vi "Image Transmission.vi"() -> ()   [LabVIEW 2013]
uses:
  <vilib>/picture/picture.llb/Draw True-Color Pixmap.vi
  <vilib>/addons/Modulation/Digital/General/MT Generate Bits (Galois, PN Order).vi
  <vilib>/addons/Modulation/Digital/General/MT Generate PSK System Parameters(M).vi
  <vilib>/addons/Modulation/Digital/General/MT Generate PSK Synchronization Parameters (bit array).vi
  <vilib>/addons/Modulation/Digital/General/MT Format Eye Diagram (complex).vi
  <vilib>/addons/Modulation/niDMT.lvlib
panel:
  in  "Tab Control":enum32{"Page 1", "Page 2"}(tab)
  out "eye diagram":cluster{"t0":dbl, "dt":dbl, "Y":dbl[]}[](graph)
  out "constellation graph":T1(graph)
  out "Recovered Image":picture
  out "Transmitted Image":picture
  in  "Path to JPEG file":path
  in  "stop":bool
  out "baseband waveform":cluster{"t0":dbl, "dt":dbl, "Y":dbl[]}(graph)
  out "LED Array":cluster{bool[], bool[]}
  out "measurements":T2 {"phase offset (deg)" format="%.2f"; "frequency drift (Hz)" format="%.2f"; "frequency offset (Hz)" format="%.2f"}
  out "sync found index (symbols)":dbl format="%.4f"
  in  "Eb/N0 (10 dB)":dbl(slide)=10.0 scale=0.0..50.0
  in  "modulation type":T3(ring)
  in  "pulse shaping filter (none)":T4(ring)
  in  "M-FSK (4)":i32=2 caption="M-FSK (2)"
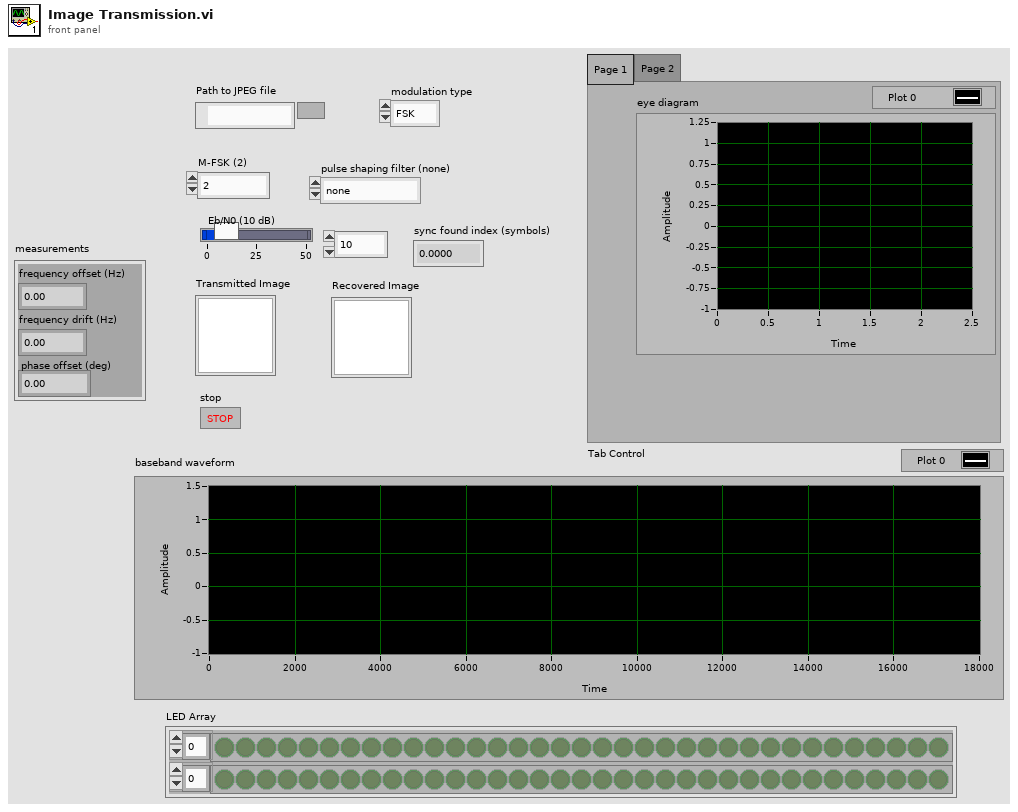
[diagram p1: front panel]
types:
  T1 = cluster{"constellation":dbl[], "oversampled data":dbl[]}[]
  T2 = cluster{"frequency offset (Hz)":dbl, "frequency drift (Hz)":dbl, "phase offset (deg)":dbl}
  T3 = enum16{"FSK", "PSK", "QAM", "MSK", "PAM", "ASK", "CPM"}
  T4 = enum16{"none", "Raised Cosine", "Root Raised Cos", "Gaussian"}
  T5 = typedef "imagedata.ctl" = cluster{"image type":i32, "image depth":i32, "image":u8[], "mask":u8[], "colors":u32[], "Rectangle":cluster{"left":i16, "top":i16, "right":i16, "bottom":i16}}
  T6 = cluster{"samples per symbol (16)":i32, "symbol map":cdb[], "differential PSK":enum16{"disable", "enable"}, "PSK type":u16}
  T7 = typedef "niAMT.lvlib/Complex Data Waveform.ctl" = cluster{"t0":dbl, "dt":dbl, "Y":cdb[]}
  T8 = cluster{"expected sync location (symbols)":i32, "sync sequence":cdb[], "sync location uncertainty (symbols)":i32, "sync indent (symbols)":i32}
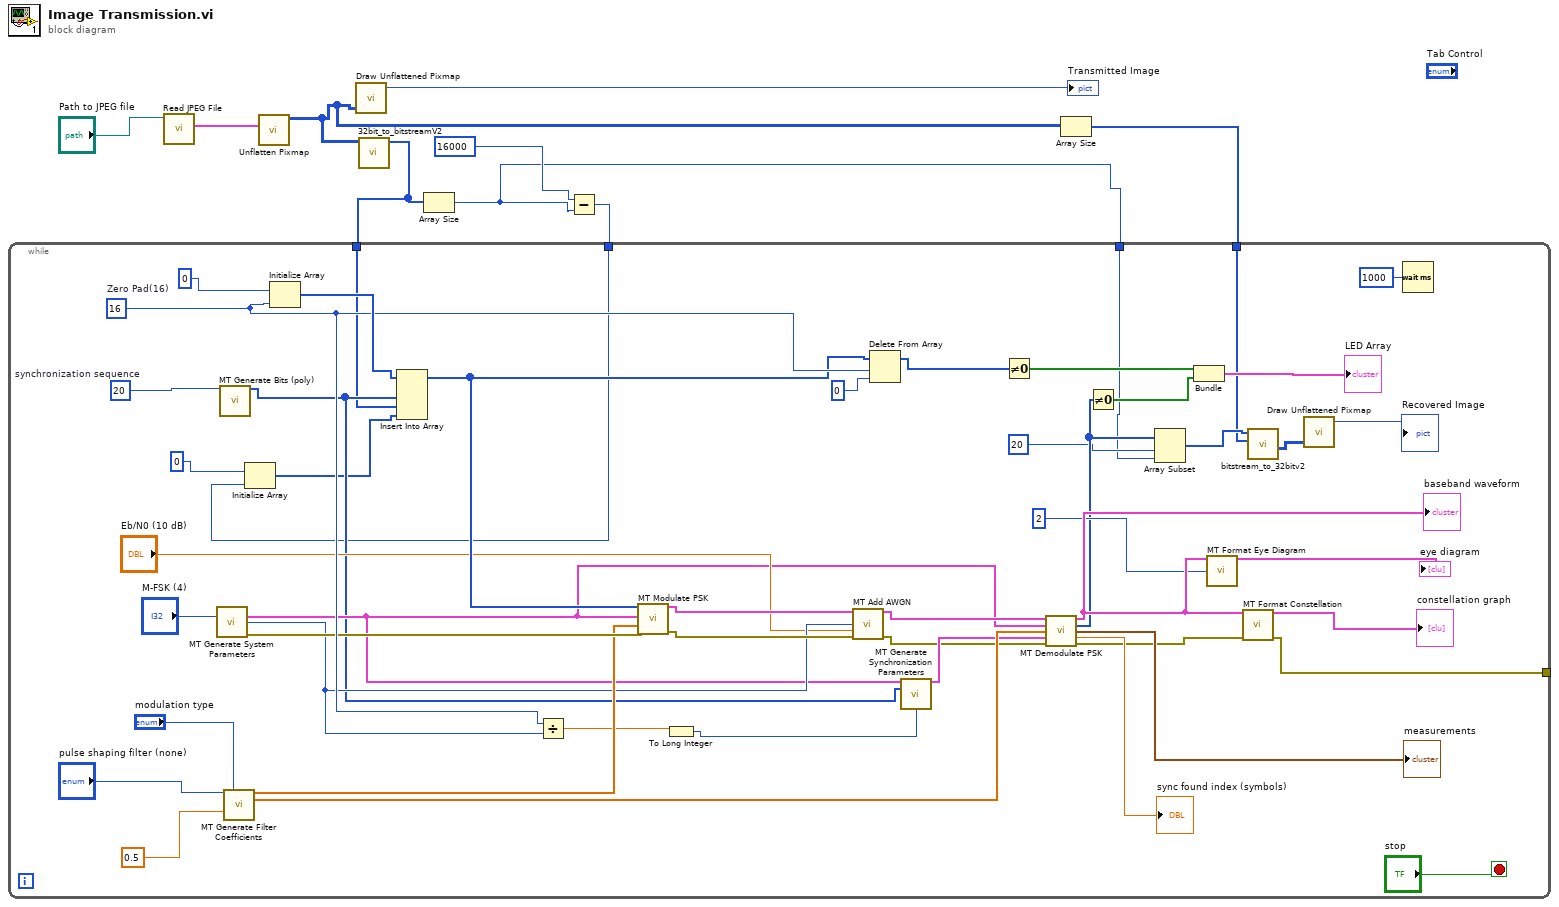
[diagram p0: block diagram]
diagram:
  n1 = call <vilib>:"Read JPEG File.vi"("path to JPEG file"="Path to JPEG file") -> ("image data"=w8:T5)  [unwired: 8 in, 2 out]
  n2 = call <vilib>:"Unflatten Pixmap.vi"("image data"=w8) -> ("24-bit pixmap"=w6:u32[][])  [unwired: 4 in, 6 out]
  n3 = call-poly <vilib>:"Draw Unflattened Pixmap.vi"("data (RGB format)"=w6) -> ("new picture"=→"Transmitted Image":picture)  [unwired: 8 in]
  n4 = call "32bit_to_bitstreamV2.vi"("24-bit pixmap"=w6) -> ("Bitstream with Guard"=w3:u8[])  [unwired: 7 in, 1 out]
  n5 = Array Size(array=w3) -> (size(s)=w2:i32)
  n6 = Subtract(x=16000, y=w2) -> (x-y=w4:i32)
  n7 = Array Size(array=w6) -> (size(s)=w1:i32[])
  n8 = while {
    tunnel: [w22] -> _
    tunnel: w4 -> [w19]
    tunnel: w3 -> [w17]
    tunnel: w2 -> [w14]
    tunnel: w1 -> [w12]
    stop <- "stop" stop-if-true
    w56 = 20  # synchronization sequence
    w47 = 16  # Zero Pad(16)
    n9 = call-poly <vilib>:"MT Generate System Parameters.vi"("M-PSK (4)"="M-FSK (4)") -> ("PSK system parameters"=w35:T6, "bits per symbol"=w41:i32, "error out"=w46:errorcluster)  [unwired: 12 in]
    n10 = call-poly <vilib>:"MT Generate Bits (poly).vi"("total bits (128)"=w56) -> ("output bit stream"=w34:i8[])  [unwired: 12 in, 2 out]
    n11 = call <vilib>:"MT Generate Filter Coefficients.vi"("pulse shaping filter (none)"="pulse shaping filter (none)", "modulation type"="modulation type", "filter parameter"=0.5) -> ("pulse shaping filter coefficients"=w45:dbl[], "matched filter coefficients"=w38:dbl[])  [unwired: 10 in, 1 out]
    n12 = Initialize Array "Initialize Array"(0, w19) -> (w18:i32[])
    n13 = Initialize Array "Initialize Array"(0, w47) -> (w57:i32[])
    n14 = Insert Into Array "Insert Into Array"(array=w57, new element #1=w34, new element #2=w17, new element #3=w18) -> (w43:i32[])  [unwired: 1 in]
    n15 = Divide(x=w47, y=w41) -> (x/y=w37:dbl)
    n16 = call <vilib>:"MT Modulate PSK.vi"("input bit stream"=w43, "PSK system parameters"=w35, "pulse shaping filter coefficients"=w45, "error in (no error)"=w46) -> ("output complex waveform"=w44:T7, "error out"=w42:errorcluster)  [unwired: 9 in, 1 out]
    n17 = To Long Integer(number=w37) -> (32bit integer=w36:i32)
    n18 = call <vilib>:"MT Add AWGN.vi"("input complex waveform"=w44, "bits per symbol (1)"=w41, "Eb/N0 (10 dB)"="Eb/N0 (10 dB)", "error in (no error)"=w42) -> ("output complex waveform"=w39:T7, "error out"=w32:errorcluster)  [unwired: 9 in, 1 out]
    n19 = Delete From Array "Delete From Array"(array=w43, length=w47, index=0) -> (array with subset deleted=w54:i32[])  [unwired: 1 out]
    n20 = call-poly <vilib>:"MT Generate Synchronization Parameters.vi"("PSK system parameters"=w35, "sync bits"=w34, "sync location uncertainty (symbols)"=w36) -> ("PSK synchronization parameters"=w33:T8)  [unwired: 11 in, 1 out]
    n21 = Not Equal To 0?(x=w54) -> (x != 0?=w53:bool[])
    n22 = call <vilib>:"MT Demodulate PSK.vi"("input complex waveform"=w39, "PSK system parameters"=w35, "matched filter coefficients"=w38, "synchronization parameters"=w33, "error in (no error)"=w32) -> ("recovered complex waveform"=w25:T7, "output bit stream"=w16:i8[], "measurements"=→"measurements":T2, "sync found index (symbols)"=→"sync found index (symbols)":dbl, "error out"=w29:errorcluster)  [unwired: 6 in]
    "baseband waveform" <- w25
    n23 = Not Equal To 0?(x=w16) -> (x != 0?=w27:bool[])
    n24 = Array Subset "Array Subset"(array=w16, index=20, length=w14) -> (w13:i8[])
    n25 = Bundle "Bundle"(w53, w27) -> (→"LED Array":cluster{bool[], bool[]})  [unwired: 1 in]
    n26 = call-poly <vilib>:"MT Format Eye Diagram.vi"("waveform"=w25, "eye length"=2) -> ("eye diagram"=→"eye diagram":cluster{"t0":dbl, "dt":dbl, "Y":dbl[]}[])  [unwired: 12 in, 1 out]
    n27 = call <vilib>:"MT Format Constellation.vi"("waveform"=w25, "error in (no error)"=w29) -> ("constellation graph"=→"constellation graph":T1, "error out"=w22:errorcluster)  [unwired: 12 in]
    n28 = call "bitstream_to_32bitv2.vi"("JPG Size"=w12, "Bitstream Input"=w13) -> ("2D JPG Array"=w11:u32[][])  [unwired: 8 in, 1 out]
    n29 = call-poly <vilib>:"Draw Unflattened Pixmap.vi"("data (RGB format)"=w11) -> ("new picture"=→"Recovered Image":picture)  [unwired: 8 in]
    n30 = Wait (ms)(milliseconds to wait=u32 1000) -> ()  [unwired: 1 out]
  }
